vi "trigger.vi"(7 "TOL":sgl format="%#_13g", 8 "Vo":sgl format="%#_13g", 11 "e(k)":sgl format="%#_13g") -> (2 "trigger":bool)   [LabVIEW 2015]
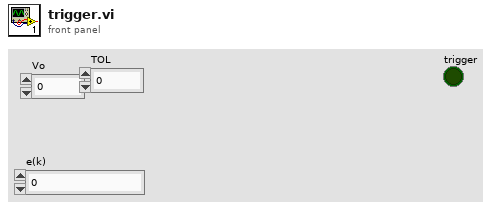
[diagram p1: front panel]
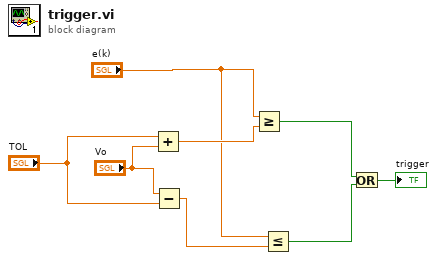
[diagram p0: block diagram]
diagram:
  n1 = Add(x="TOL", y="Vo") -> (x+y=w6:sgl)
  n2 = Subtract(x="Vo", y="TOL") -> (x-y=w4:sgl)
  n3 = Greater Or Equal?(x="e(k)", y=w6) -> (x >= y?=w3:bool)
  n4 = Less Or Equal?(x="e(k)", y=w4) -> (x <= y?=w2:bool)
  n5 = Or(x=w3, y=w2) -> (x .or. y?=→"trigger":bool)
